vi "LookAheadPoint.vi"(6 "Reset":bool, 8 "Robot":cluster{"x":dbl, "y":dbl}, 9 "Spacing":dbl, 10 "LookAhead":dbl, 11 "Path":cluster{"x":dbl, "y":dbl}[](array[cluster])) -> (2 "LookaheadIndex":i32, 3 "Point":cluster{"x":dbl, "y":dbl})   [LabVIEW 2019]
doc: "Finds the lookahead point given a path and the current location of the robot."
panel:
  out "t":dbl
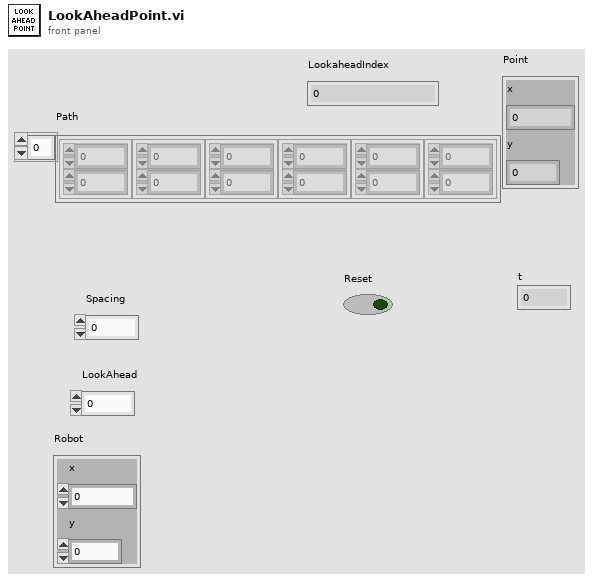
[diagram p1: front panel]
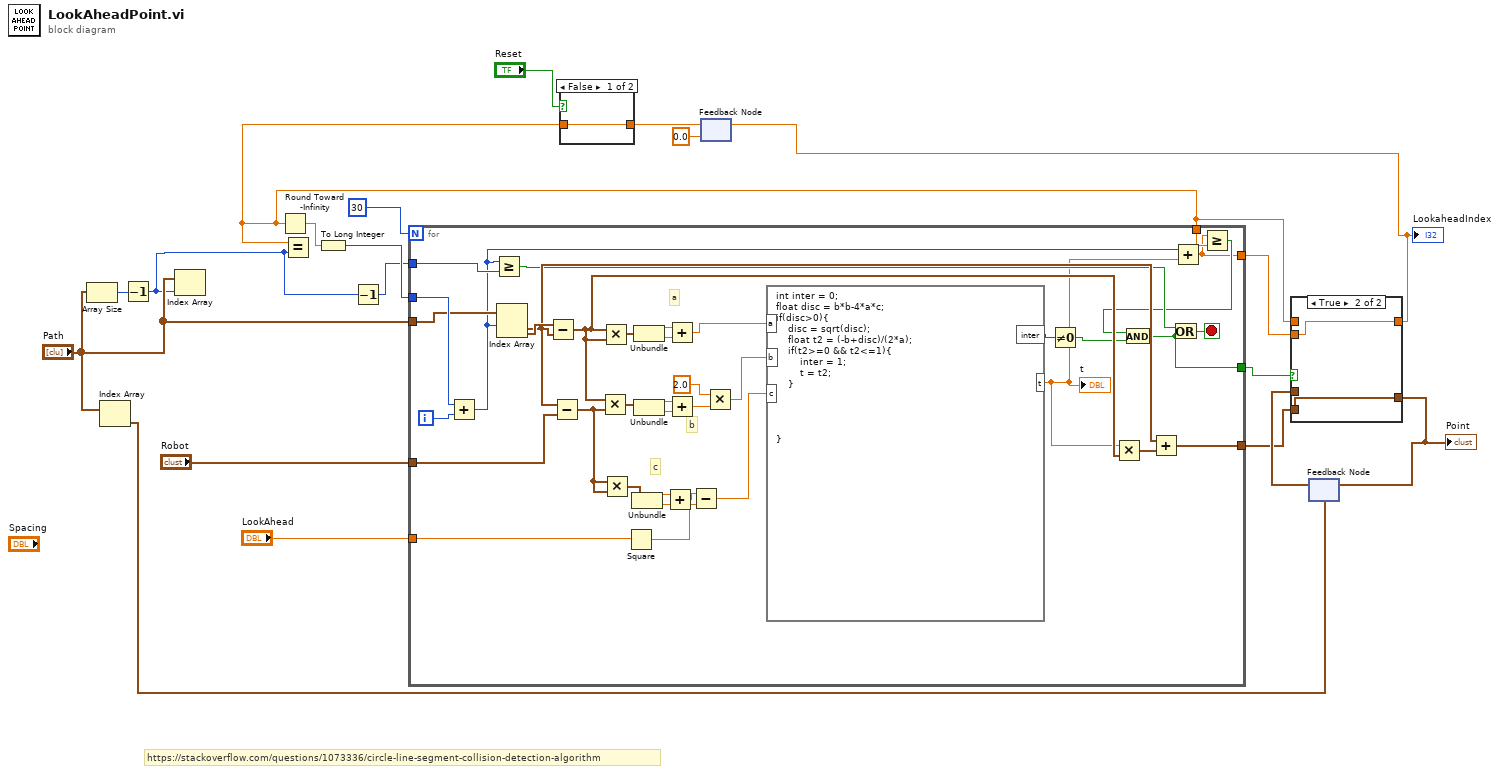
[diagram p0: block diagram]
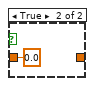
[diagram p3: hidden frame]
diagram:
  # "https://stackoverflow.com/questions/1073336/circle-line-segment-collision-detection-algorithm"
  n1 = Array Size(array="Path") -> (size(s)=w20:i32)
  n2 = Index Array(array="Path") -> (element=w11:cluster{"x":dbl, "y":dbl})  [unwired: 1 in]
  n3 = Decrement(x=w20) -> (x-1=w3:i32)
  n4 = Index Array(array="Path", index=w3) -> ()  [unwired: 1 out]
  n5 = Decrement(x=w3) -> (x-1=w2:i32)
  n6 = feedback #1(0.0) -> (w18:dbl)
  n7 = case shown="False" "Reset" {
    tunnel: w18 -> [w21 _]
    tunnel: [w21 0.0] -> w1
    frame False {
    }
    frame True {
    }
  }
  n8 = Round Toward -Infinity(1:w1) -> (0:w5:dbl)
  n9 = Equal?(x=w1, y=w3) -> ()  [unwired: 1 out]
  n10 = To Long Integer(number=w5) -> (32bit integer=w7:i32)
  n11 = for {
    N: 30 -> [_]
    tunnel: w7 -> [w59]
    tunnel: "Path" -> [w58]
    tunnel: "Robot" -> [w57]
    tunnel: "LookAhead" -> [w53]
    tunnel: [w45] -> w9
    tunnel: [w23] -> w8
    tunnel: [w27] -> w14
    tunnel: w2 -> [w30]
    tunnel: w1 -> [w25]
    i -> [w60]
    stop <- w32 stop-if-true
    # "c"
    # "b"
    # "a"
    n12 = Add(x=w59, y=w60) -> (x+y=w29:i32)
    n13 = Greater Or Equal?(x=w29, y=w30) -> (x >= y?=w31:bool)
    n14 = Index Array(array=w58, index #1=w29) -> (element #1=w46:cluster{"x":dbl, "y":dbl}, element #2=w47:cluster{"x":dbl, "y":dbl})  [unwired: 1 in]
    n15 = Subtract(x=w47, y=w46) -> (x-y=w49:cluster{"x":dbl, "y":dbl})
    n16 = Subtract(x=w46, y=w57) -> (x-y=w55:cluster{"x":dbl, "y":dbl})
    n17 = Multiply(x=w49, y=w55) -> (x*y=w38:cluster{"x":dbl, "y":dbl})
    n18 = Multiply(x=w49, y=w49) -> (x*y=w44:cluster{"x":dbl, "y":dbl})
    n19 = Multiply(x=w55, y=w55) -> (x*y=w34:cluster{"x":dbl, "y":dbl})
    n20 = Square(x=w53) -> (x^2=w54:dbl)
    n21 = Unbundle(w34) -> ("x"=w35:dbl, "y"=w36:dbl)
    n22 = Unbundle(w44) -> ("x"=w42:dbl, "y"=w43:dbl)
    n23 = Unbundle(w38) -> ("x"=w39:dbl, "y"=w40:dbl)
    n24 = Add(x=w35, y=w36) -> (x+y=w33:dbl)
    n25 = Add(x=w42, y=w43) -> (x+y=w41:dbl)
    n26 = Add(x=w39, y=w40) -> (x+y=w37:dbl)
    n27 = Subtract(x=w33, y=w54) -> (x-y=w51:dbl)
    n28 = Multiply(x=2.0, y=w37) -> (x*y=w52:dbl)
    n29 = formula code="int inter = 0;\nfloat disc = b*b-4*a*c;\nif(disc>0){\n    disc = sqrt(disc);\n    float t2 = (-b+disc)/(2*a);\n    if(t2>=0 && t2<=1){\n        inter = 1;\n        t = t2;\n    }\n\n\n\n\n}"("a"=w41, "b"=w52, "c"=w51) -> ("inter"=w50:i32, "t"=w26:dbl)
    "t" <- w26
    n30 = Not Equal To 0?(x=w50) -> (x != 0?=w28:bool)
    n31 = Multiply(x=w26, y=w49) -> (x*y=w48:cluster{"x":dbl, "y":dbl})
    n32 = Add(x=w46, y=w48) -> (x+y=w45:cluster{"x":dbl, "y":dbl})
    n33 = Add(x=w29, y=w26) -> (x+y=w23:dbl)
    n34 = Greater Or Equal?(x=w23, y=w25) -> (x >= y?=w24:bool)
    n35 = And(x=w24, y=w28) -> (x .and. y?=w27:bool)
    n36 = Or(x=w31, y=w27) -> (x .or. y?=w32:bool)
  }
  n37 = feedback #2(w11) -> (w13:cluster{"x":dbl, "y":dbl})
  n38 = case shown="True" w14 {
    tunnel: w13 -> [w62 _]
    tunnel: [w62 w64] -> w10
    tunnel: w9 -> [_ w64]
    tunnel: w8 -> [_ w63]
    tunnel: w1 -> [w61 _]
    tunnel: [w61 w63] -> w6
    frame False {
    }
    frame True {
    }
  }
  "Point" <- w10
  "LookaheadIndex" <- w6
  n39 = feedback-in #1(w6) -> ()
  n40 = feedback-in #2(w10) -> ()
